vi "Program Blank Device.vi"(0 "State-machine Local Variables":T1={"Message"="", "Homed?"=FALSE, "NextState"=enum."Timeout", "G.Load"=0.0, "G.Position"=0.0, "Load#"=0, "[G.Loads]"=[], "[TotalLoads]"=[], "[Errors]"=[], "ZeroWait"=0, "Results"=[], "DwellWait"=FALSE, "Test Result"=FALSE, "[CondyleLoads]"=[], "[Max]"=[], "[Min]"=[], "Valid String?"=FALSE, "ScanTime"=timestamp(0 s since 1904-01-01), "ScannedString"="", "LabelDevID"=0, "MfgDate"=timestamp(0 s since 1904-01-01), "[EEPROM Cmds]"=[], "[CalData]"=[], "[A/Ds]"=[], "[A/Dmax]"=[], "[A/Dmin]"=[], "BattMax"=0.0, "BattMin"=0.0, "DwellTime"=2000, "PendingDeviceType"="", "Zero G.load"=0.0, "GAINC Value"="", "Programming Step"=enum."Load EEPROM", "Front Panel Program?"=FALSE, "Final Program?"=FALSE, "PCB Score"=100, "AssyScore"=100, "Pass/Fail #"="", "Result String"="", "Programming Mode"=enum."Initial Program", "Angle Test Step"=enum."Initialize", "Accel Values"=[], "Shutdown Counter"=0, "V1"=0, "V2"=0, "V3"=0, "V4"=0, "EEPROM Data"=[], "Counter"=0, "Page#"=0, "Timer"=timestamp(0 s since 1904-01-01), "Use Mark10?"=FALSE, "Eng-Result#"=0, "DUT Serial #"=0, "Scroll Message?"=FALSE, "Clear Message"=FALSE, "Batt Test Step "=enum."Initialize", "RXTX Window Found?"=FALSE, "Shutdown First Call?"=FALSE, "A2 Delay (msec)"=500, "Support Script"={"Script #"="", "Script Revision"="", "[OEMs]"=[], "[[DeviceTypes]]"=[], "[[DeviceTypesVals]]"=[], "[[List of Errors]]"=[], "Default GAINC"="", "[[ASICtrims]]"=[], "ID For Echo"="", "Condyle A CalFactor"=100, "Condyle B CalFactor"=100, "[OEMs Prefix]"=[], "Packet ID 18"="", "[[Force Table Load Test]]"=[], "[[Force Table AccurTest]]"=[]}, "Serial Table"={"Serial File Path"=path "", "[[Serial Lookup Table]]"=[], "Serial Device Info"=[], "Valid Serial?"=FALSE}, "Target Information"={"Target Brand"="", "Target DeviceType"="", "Target Serial#"=100, "Target Lot#"=0, "Target DevID"=0, "Target Channel"=5}, "Operator"="", "COM Port"="", "Config Path"=path "", "Tx Array"=[], "DUT Parameters"={"Channel"=0, "DeviceID"=0, "Script Rev"=0, "Month"=0, "Day"=0, "Year"=0, "Lot#"=0, "V1"=0, "V2"=0, "V3"=0, "V4"=0, "MFG"=0, "Cal FactorA 10"=0, "Cal FactorB 10  "=0, "Cal FactorA 16"=0, "Cal FactorB 16"=0, "ASICtrim"=[], "TmpChan"=0, "GAINC"="", "Brand"="", "Device"="", "Serial #"=0, "Batt310"=0, "Batt 280"=0}, "FTS Main?"=FALSE, "Loading"={"[Forces]"=[], "[Dwell]"=[], "Loading Step"=enum."Initialize Test"}, "Software Version"="", "Correction Factor"="", "Second Load Test"=FALSE, "Acc Loads"=[], "Mark10 Config"={"H2S%"=[80.0, 85.0, 90.0, 95.0, 100.0], "H2S Speed"=[12.0, 8.0, 6.0, 4.0, 2.0], "H to S"=2.0, "Home Speed"=1.0, "LoadWin"=0.0, "Load Speed"=0.0, "PID"={"Kp"=0.04, "Kd"=0.005001, "Ki"=2.9999999999999923e-05}}, "Channels"={"Transceiver Ch"=5, "Operating Ch"=5, "Start Ch"=0}, "Channel EEPROM"=[], "Load Notes"=[], "Engr Log?"=FALSE, "Time"=[], "Program Retry"=FALSE, "Operator Channel"="", "Target Channel "="", "New Data Program"=FALSE, "NFHU Pass?"=FALSE, "Cycle Number"=0, "Cal Cycle#"=0, "[Avg G.Loads] "=[], "[Avg A/Ds] "=[], "Cal Retry?"=FALSE, "[Total A/Ds]  "=[], "Cycle Num LA"=0, "LA Cycle# "=0, "Shim Num"=0, "Shim#  "=0, "Angle Test?"=FALSE} {"Mark10 Config"."PID"."Ki" min=0.0 max=200.0 format="%.6f"; "Mark10 Config"."PID"."Kd" min=0.0 max=200.0 format="%.6f"; "Mark10 Config"."PID"."Kp" min=0.0 max=200.0 format="%.6f"; "DUT Parameters"."ASICtrim" format="%02x"}, 11 "error in (no error)":errorcluster) -> (4 "State-machine Local Variables 2":T1={"Message"="", "Homed?"=FALSE, "NextState"=enum."Timeout", "G.Load"=0.0, "G.Position"=0.0, "Load#"=0, "[G.Loads]"=[], "[TotalLoads]"=[], "[Errors]"=[], "ZeroWait"=0, "Results"=[], "DwellWait"=FALSE, "Test Result"=FALSE, "[CondyleLoads]"=[], "[Max]"=[], "[Min]"=[], "Valid String?"=FALSE, "ScanTime"=timestamp(0 s since 1904-01-01), "ScannedString"="", "LabelDevID"=0, "MfgDate"=timestamp(0 s since 1904-01-01), "[EEPROM Cmds]"=[], "[CalData]"=[], "[A/Ds]"=[], "[A/Dmax]"=[], "[A/Dmin]"=[], "BattMax"=0.0, "BattMin"=0.0, "DwellTime"=2000, "PendingDeviceType"="", "Zero G.load"=0.0, "GAINC Value"="", "Programming Step"=enum."Load EEPROM", "Front Panel Program?"=FALSE, "Final Program?"=FALSE, "PCB Score"=100, "AssyScore"=100, "Pass/Fail #"="", "Result String"="", "Programming Mode"=enum."Initial Program", "Angle Test Step"=enum."Initialize", "Accel Values"=[], "Shutdown Counter"=0, "V1"=0, "V2"=0, "V3"=0, "V4"=0, "EEPROM Data"=[], "Counter"=0, "Page#"=0, "Timer"=timestamp(0 s since 1904-01-01), "Use Mark10?"=FALSE, "Eng-Result#"=0, "DUT Serial #"=0, "Scroll Message?"=FALSE, "Clear Message"=FALSE, "Batt Test Step "=enum."Initialize", "RXTX Window Found?"=FALSE, "Shutdown First Call?"=FALSE, "A2 Delay (msec)"=500, "Support Script"={"Script #"="", "Script Revision"="", "[OEMs]"=[], "[[DeviceTypes]]"=[], "[[DeviceTypesVals]]"=[], "[[List of Errors]]"=[], "Default GAINC"="", "[[ASICtrims]]"=[], "ID For Echo"="", "Condyle A CalFactor"=100, "Condyle B CalFactor"=100, "[OEMs Prefix]"=[], "Packet ID 18"="", "[[Force Table Load Test]]"=[], "[[Force Table AccurTest]]"=[]}, "Serial Table"={"Serial File Path"=path "", "[[Serial Lookup Table]]"=[], "Serial Device Info"=[], "Valid Serial?"=FALSE}, "Target Information"={"Target Brand"="", "Target DeviceType"="", "Target Serial#"=100, "Target Lot#"=0, "Target DevID"=0, "Target Channel"=5}, "Operator"="", "COM Port"="", "Config Path"=path "", "Tx Array"=[], "DUT Parameters"={"Channel"=0, "DeviceID"=0, "Script Rev"=0, "Month"=0, "Day"=0, "Year"=0, "Lot#"=0, "V1"=0, "V2"=0, "V3"=0, "V4"=0, "MFG"=0, "Cal FactorA 10"=0, "Cal FactorB 10  "=0, "Cal FactorA 16"=0, "Cal FactorB 16"=0, "ASICtrim"=[], "TmpChan"=0, "GAINC"="", "Brand"="", "Device"="", "Serial #"=0, "Batt310"=0, "Batt 280"=0}, "FTS Main?"=FALSE, "Loading"={"[Forces]"=[], "[Dwell]"=[], "Loading Step"=enum."Initialize Test"}, "Software Version"="", "Correction Factor"="", "Second Load Test"=FALSE, "Acc Loads"=[], "Mark10 Config"={"H2S%"=[80.0, 85.0, 90.0, 95.0, 100.0], "H2S Speed"=[12.0, 8.0, 6.0, 4.0, 2.0], "H to S"=2.0, "Home Speed"=1.0, "LoadWin"=0.0, "Load Speed"=0.0, "PID"={"Kp"=0.04, "Kd"=0.005001, "Ki"=2.9999999999999923e-05}}, "Channels"={"Transceiver Ch"=5, "Operating Ch"=5, "Start Ch"=0}, "Channel EEPROM"=[], "Load Notes"=[], "Engr Log?"=FALSE, "Time"=[], "Program Retry"=FALSE, "Operator Channel"="", "Target Channel "="", "New Data Program"=FALSE, "NFHU Pass?"=FALSE, "Cycle Number"=0, "Cal Cycle#"=0, "[Avg G.Loads] "=[], "[Avg A/Ds] "=[], "Cal Retry?"=FALSE, "[Total A/Ds]  "=[], "Cycle Num LA"=0, "LA Cycle# "=0, "Shim Num"=0, "Shim#  "=0, "Angle Test?"=FALSE} {"Mark10 Config"."PID"."Ki" min=0.0 max=200.0 format="%.6f"; "Mark10 Config"."PID"."Kd" min=0.0 max=200.0 format="%.6f"; "Mark10 Config"."PID"."Kp" min=0.0 max=200.0 format="%.6f"; "DUT Parameters"."ASICtrim" format="%02x"}, 6 "Program Successful":bool, 15 "error out":errorcluster)   [LabVIEW 2015]
uses:
  Controls/LocalVars.ctl
  Controls/Gen2 FT states.ctl
  Controls/Iniial Device Programming.ctl
  ProgramStageControl.ctl
  Controls/Batt Cap Steps.ctl
  Controls/Support Script.ctl
  Controls/Serial Table.ctl
  Controls/Device Information.ctl
  Controls/InfoPacket.ctl
  Controls/Loading.ctl
  Controls/Load Step.ctl
  Controls/Mark10 Config.ctl
  Controls/PID parameters.ctl
  Controls/Channels.ctl
  Controls/Blank Program State.ctl
  RxTx/XceiverStates.ctl
  RxTx/XceiverCmds.ctl
  Controls/Gen2 FT Globals.vi
panel:
  out "Numeric":i32
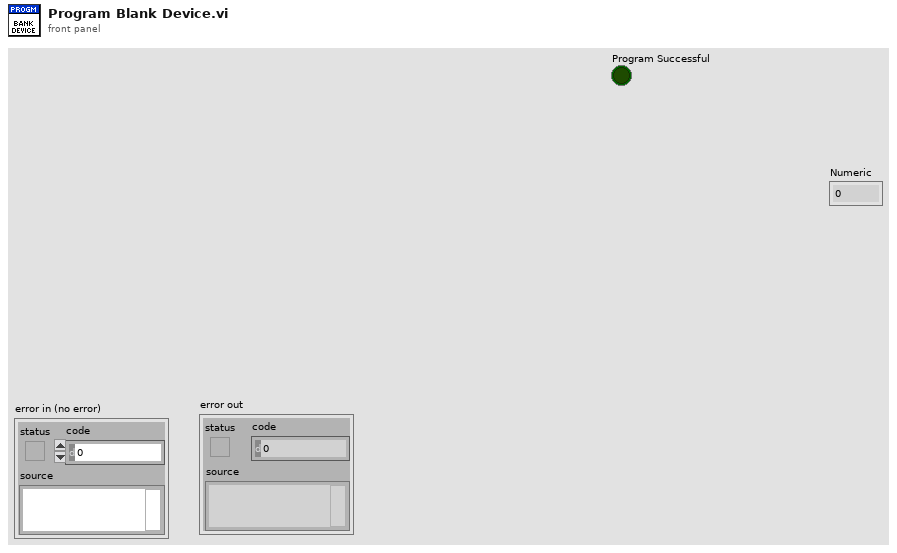
[diagram p1: front panel]
types:
  T1 = typedef "LocalVars.ctl" = cluster{"Message":string, "Homed?":bool, "NextState":T2, "G.Load":dbl, "G.Position":dbl, "Load#":i32, "[G.Loads]":dbl[], "[TotalLoads]":dbl[], "[Errors]":dbl[][], "ZeroWait":u32, "Results":dbl[], "DwellWait":bool, "Test Result":bool, "[CondyleLoads]":dbl[][], "[Max]":dbl[], "[Min]":dbl[], "Valid String?":bool, "ScanTime":timestamp, "ScannedString":string, "LabelDevID":u32, "MfgDate":timestamp, "[EEPROM Cmds]":u8[][], "[CalData]":u8[][], "[A/Ds]":dbl[][], "[A/Dmax]":dbl[], "[A/Dmin]":dbl[], "BattMax":dbl, "BattMin":dbl, "DwellTime":i32, "PendingDeviceType":string, "Zero G.load":dbl, "GAINC Value":string, "Programming Step":T3, "Front Panel Program?":bool, "Final Program?":bool, "PCB Score":i32, "AssyScore":i32, "Pass/Fail #":string, "Result String":string, "Programming Mode":T4, "Angle Test Step":enum16{"Initialize", "Get X", "Get Y", "Get Z", "Next Test"}, "Accel Values":dbl[][], "Shutdown Counter":u32, "V1":i32, "V2":i32, "V3":i32, "V4":i32, "EEPROM Data":i32[][], "Counter":i32, "Page#":i32, "Timer":timestamp, "Use Mark10?":bool, "Eng-Result#":u32, "DUT Serial #":i32, "Scroll Message?":bool, "Clear Message":bool, "Batt Test Step ":T5, "RXTX Window Found?":bool, "Shutdown First Call?":bool, "A2 Delay (msec)":i16, "Support Script":T6, "Serial Table":T7, "Target Information":T8, "Operator":string, "COM Port":string, "Config Path":path, "Tx Array":u8[], "DUT Parameters":T9, "FTS Main?":bool, "Loading":T10, "Software Version":string, "Correction Factor":string, "Second Load Test":bool, "Acc Loads":dbl[][], "Mark10 Config":T12, "Channels":T14, "Channel EEPROM":i32[][], "Load Notes":string[], "Engr Log?":bool, "Time":timestamp[], "Program Retry":bool, "Operator Channel":string, "Target Channel ":string, "New Data Program":bool, "NFHU Pass?":bool, "Cycle Number":i32, "Cal Cycle#":i32, "[Avg G.Loads] ":dbl[], "[Avg A/Ds] ":dbl[][], "Cal Retry?":bool, "[Total A/Ds]  ":dbl[][], "Cycle Num LA":i32, "LA Cycle# ":i32, "Shim Num":i32, "Shim#  ":i32, "Angle Test?":bool}
  T2 = typedef "Gen2 FT states.ctl" = enum16{"---------SETUP-------", "Initialization", "Read Support Data", "Initialize Mark-10", "Initialize Transceiver", "------UTILITIES------", "Change DUT Channel", "Find RxTx Window", "Reset Device", "Scan Channels", "Read Serial Lookup", "Shutdown Device", "ESTOP", "--------USER---------", "Timeout", "-----PROGRAM-----", "Program Device", "------MARK10--------", "Go Home", "MoveUp", "MoveDown", "Goto Load", "Goto Position", "Stop Motor", "---------TESTS--------", "Start Test", "Angle Test", "Load Test", "Load Accuracy Test", "Battery Test", "------RESULTS-------", "End Test", "Display Result", "--------EXIT--------", "Exit"}
  T3 = typedef "Iniial Device Programming.ctl" = enum16{"Load EEPROM", "Send First A1", "Send EEPROM", "Send A1", "Check EEPROM Echo", "Verify transmission", "Programming Successful", "Programming Failed"}
  T4 = typedef "ProgramStageControl.ctl" = enum16{"Initial Program", "GainC", "Scales"}
  T5 = typedef "Batt Cap Steps.ctl" = enum16{"Initialize", "Collect 2.8 Volts", "Collect 3.1 Volts", "Check Results"}
  T6 = typedef "Support Script.ctl" = cluster{"Script #":string, "Script Revision":string, "[OEMs]":string[], "[[DeviceTypes]]":string[][], "[[DeviceTypesVals]]":u16[][], "[[List of Errors]]":string[][], "Default GAINC":string, "[[ASICtrims]]":u8[][], "ID For Echo":string, "Condyle A CalFactor":i32, "Condyle B CalFactor":i32, "[OEMs Prefix]":string[], "Packet ID 18":string, "[[Force Table Load Test]]":dbl[][], "[[Force Table AccurTest]]":dbl[][]}
  T7 = typedef "Serial Table.ctl" = cluster{"Serial File Path":path, "[[Serial Lookup Table]]":string[][], "Serial Device Info":string[], "Valid Serial?":bool}
  T8 = typedef "Device Information.ctl" = cluster{"Target Brand":string, "Target DeviceType":string, "Target Serial#":i32, "Target Lot#":u32, "Target DevID":u32, "Target Channel":u8}
  T9 = typedef "InfoPacket.ctl" = cluster{"Channel":u8, "DeviceID":u32, "Script Rev":u8, "Month":u8, "Day":u8, "Year":u8, "Lot#":u32, "V1":u16, "V2":u16, "V3":u16, "V4":u16, "MFG":u8, "Cal FactorA 10":u8, "Cal FactorB 10  ":u8, "Cal FactorA 16":u8, "Cal FactorB 16":u8, "ASICtrim":u8[], "TmpChan":u8, "GAINC":string, "Brand":string, "Device":string, "Serial #":u64, "Batt310":u16, "Batt 280":u16}
  T10 = typedef "Loading.ctl" = cluster{"[Forces]":dbl[], "[Dwell]":dbl[], "Loading Step":T11}
  T11 = typedef "Load Step.ctl" = enum16{"Initialize Test", "Go Home", "Detect Dev Surface", "Wait to zero Device", "Zero Device", "Do Test", "Test Result"}
  T12 = typedef "Mark10 Config.ctl" = cluster{"H2S%":dbl[], "H2S Speed":dbl[], "H to S":dbl, "Home Speed":dbl, "LoadWin":dbl, "Load Speed":dbl, "PID":T13}
  T13 = typedef "PID parameters.ctl" = cluster{"Kp":dbl, "Kd":dbl, "Ki":dbl}
  T14 = typedef "Channels.ctl" = cluster{"Transceiver Ch":u8, "Operating Ch":u8, "Start Ch":u8}
  T15 = typedef "Blank Program State.ctl" = enum16{"Loading EEPROM data", "Send Page 0", "Program", "Verify transmission", "Programming Successful", "Programming Failed"}
  T16 = typedef "XceiverStates.ctl" = enum16{"Initialize", "Rx", "Tx", "Raw Mode", "Clear Buffer", "ClearEcho", "Read Buffer", "Close"}
  T17 = typedef "XceiverCmds.ctl" = enum8{"Get Window", "Set Window", "Load&Xmit", "Find Window", "Load CC1101", "Blink LED1", "Blink LED2", "Gen2 Mode", "Request Rev", "Gen2 Mode & Req Rev", "Load Device Settings", "Reset Xceiver", "Set Channel", "Read Channel"}
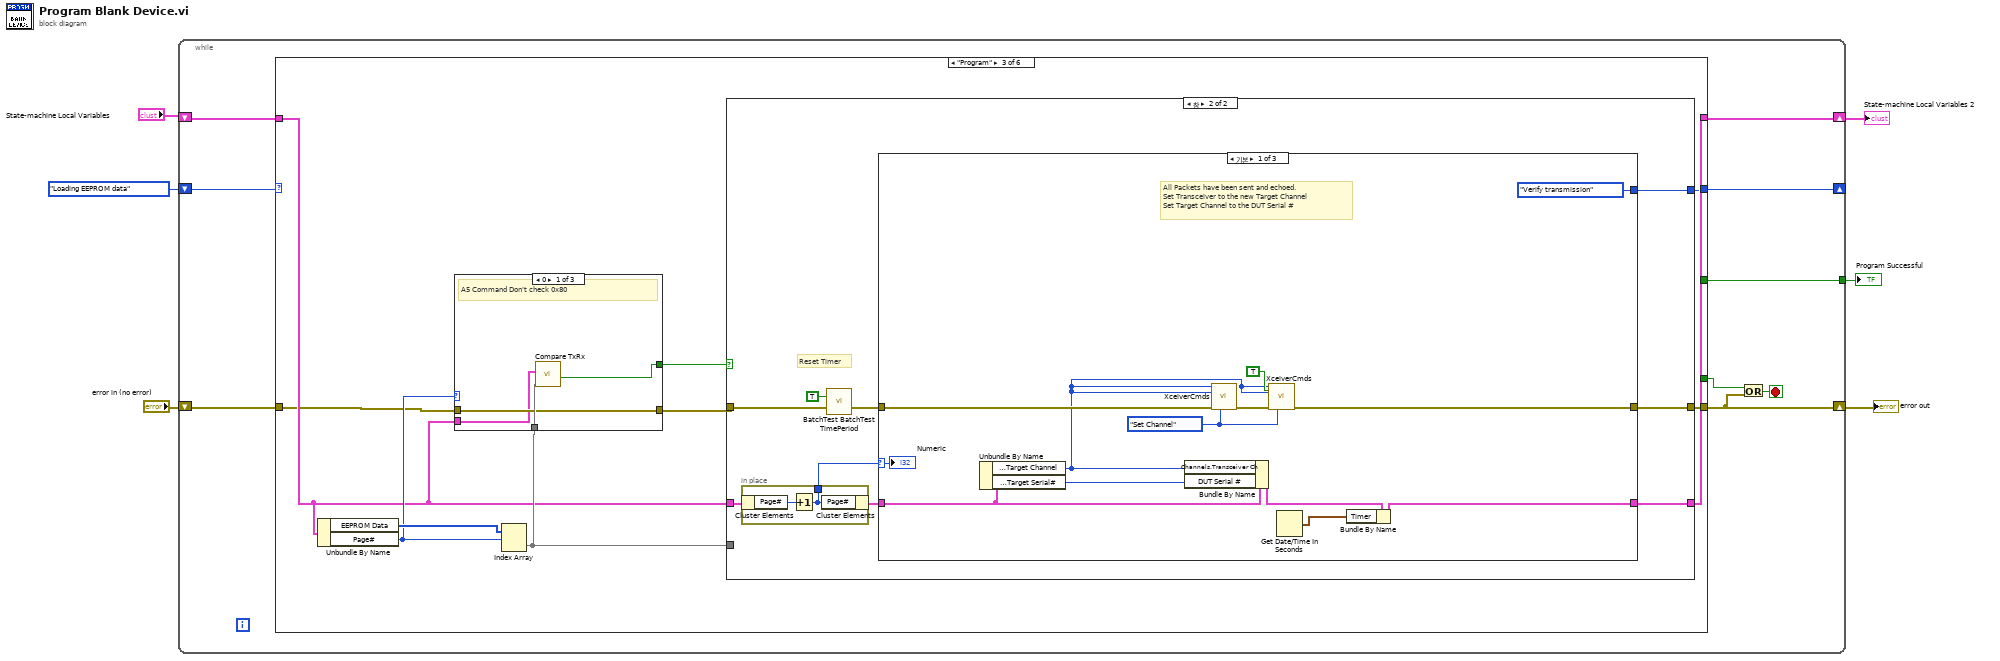
[diagram p0: block diagram]
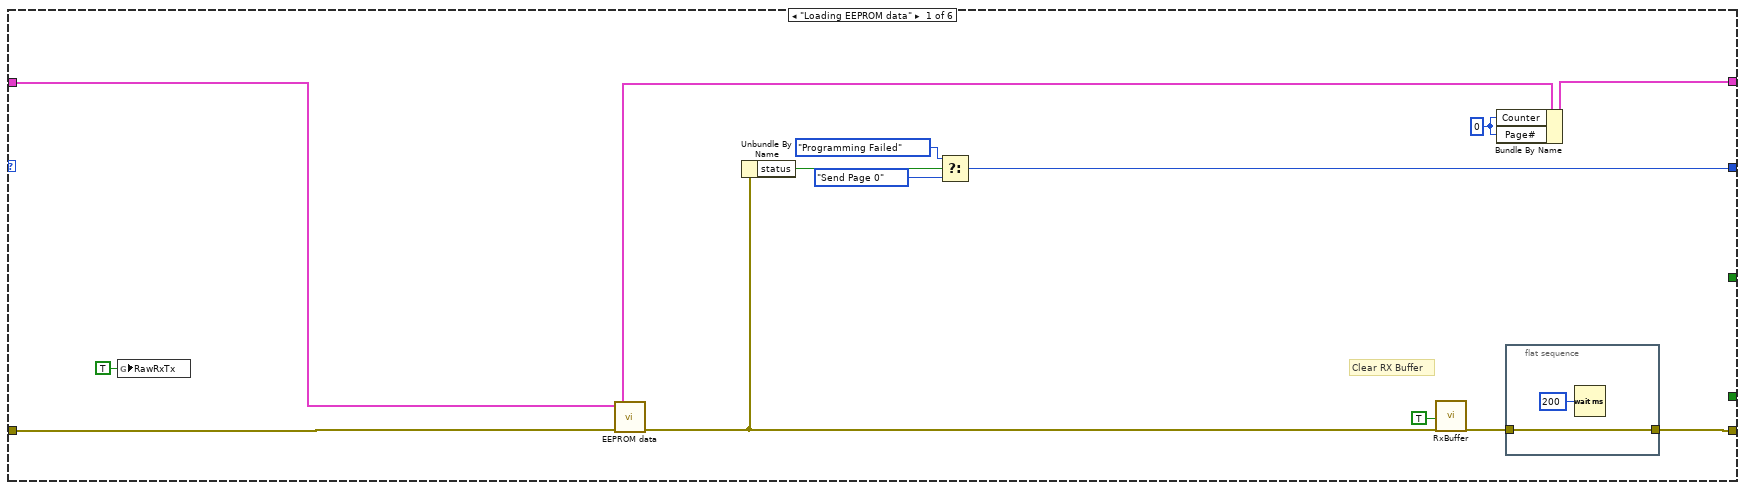
[diagram p2: hidden frame]
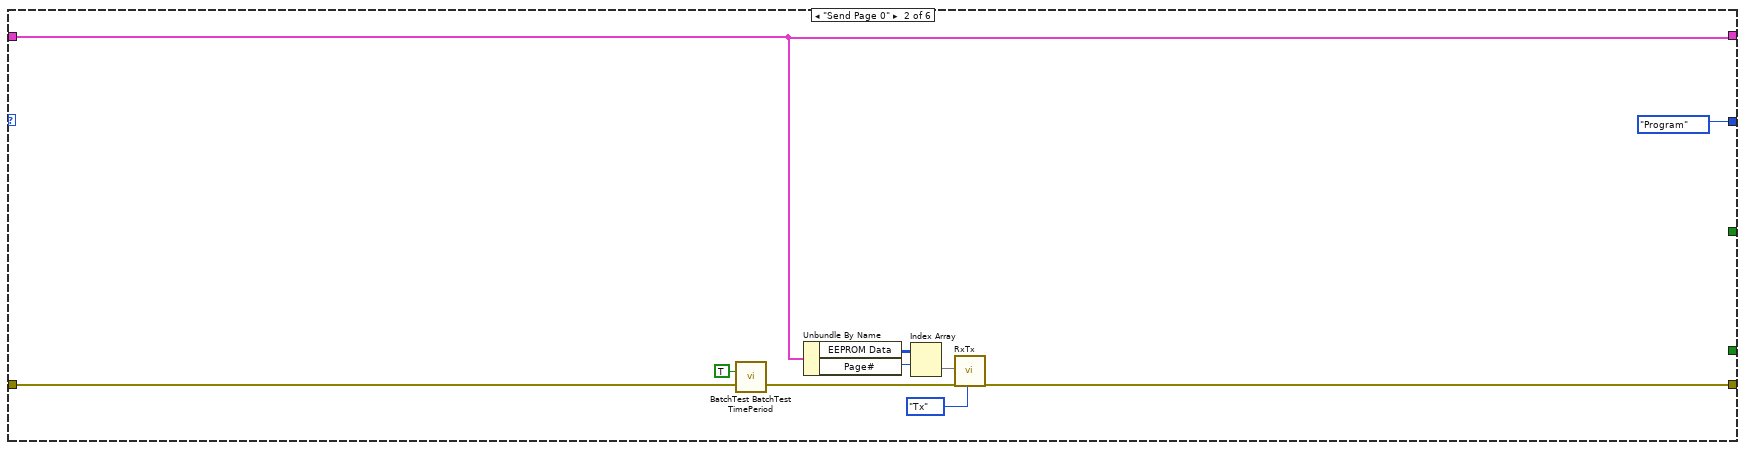
[diagram p3: hidden frame]
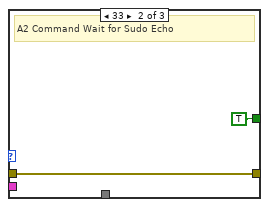
[diagram p4: hidden frame]
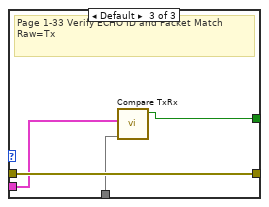
[diagram p5: hidden frame]
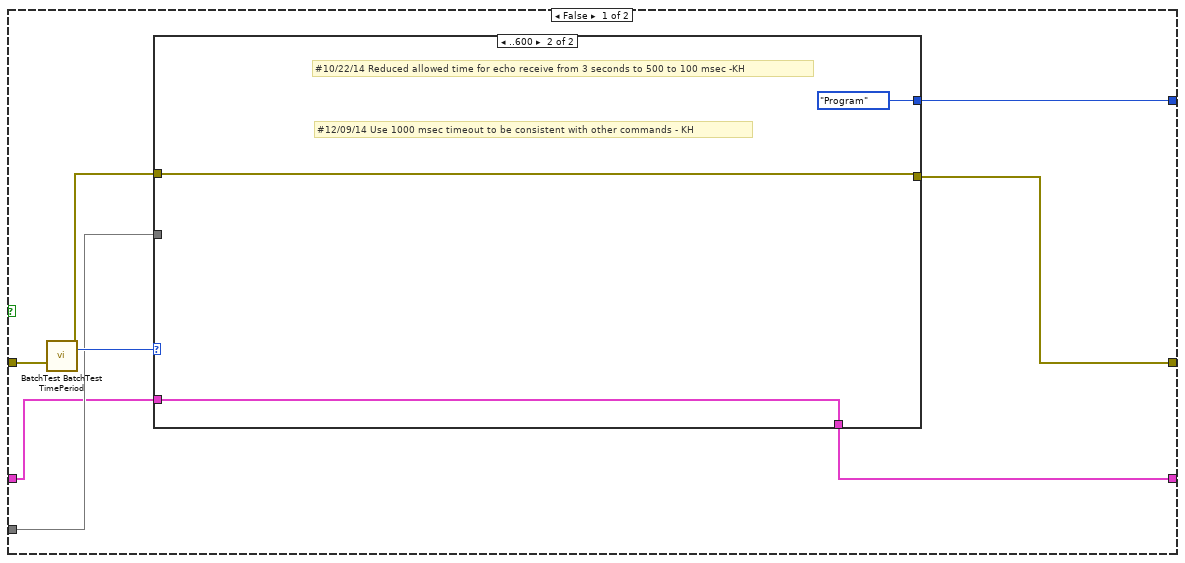
[diagram p6: hidden frame]
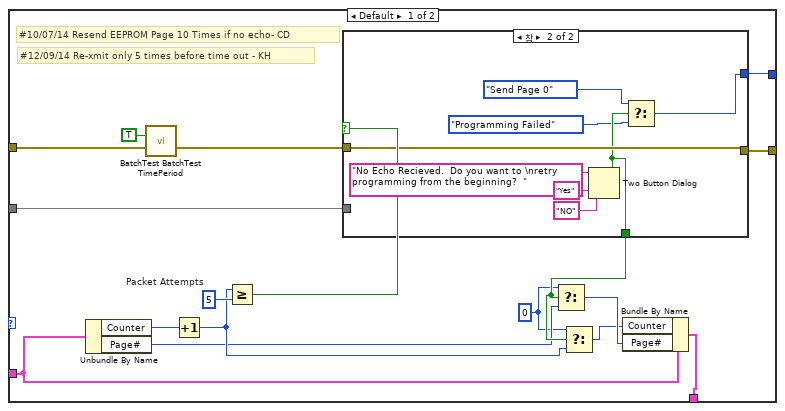
[diagram p7: hidden frame]
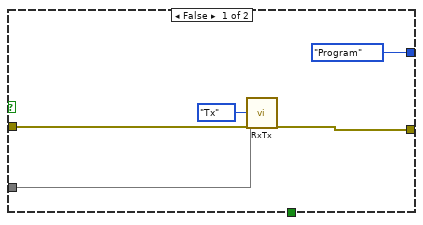
[diagram p8: hidden frame]
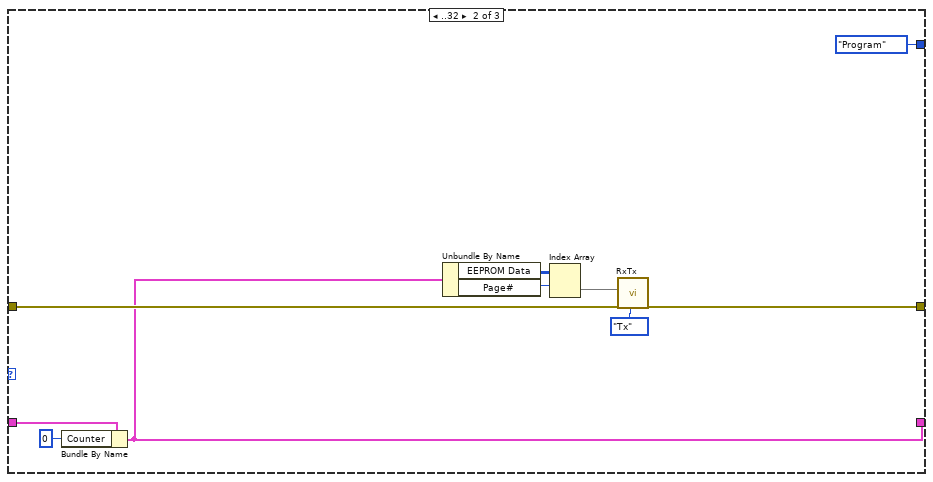
[diagram p9: hidden frame]
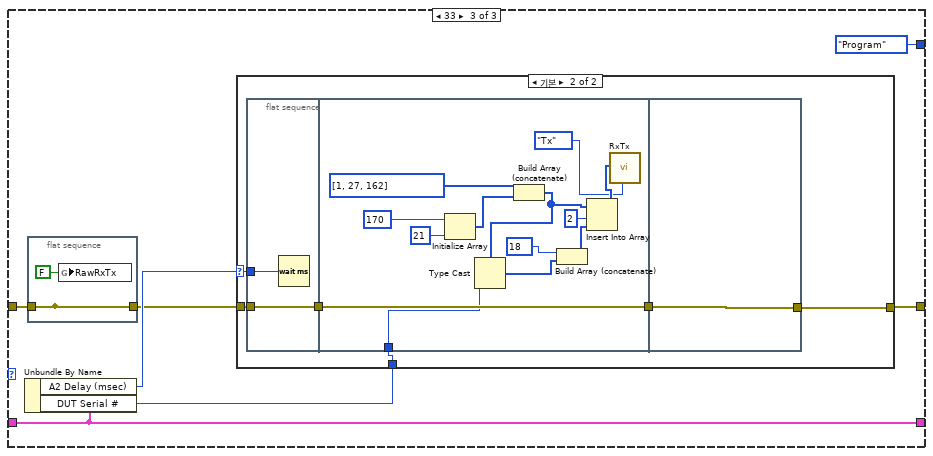
[diagram p10: hidden frame]
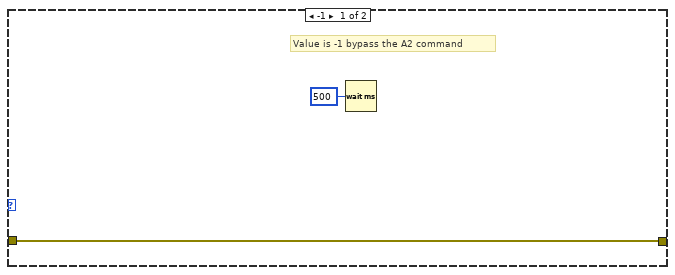
[diagram p11: hidden frame]
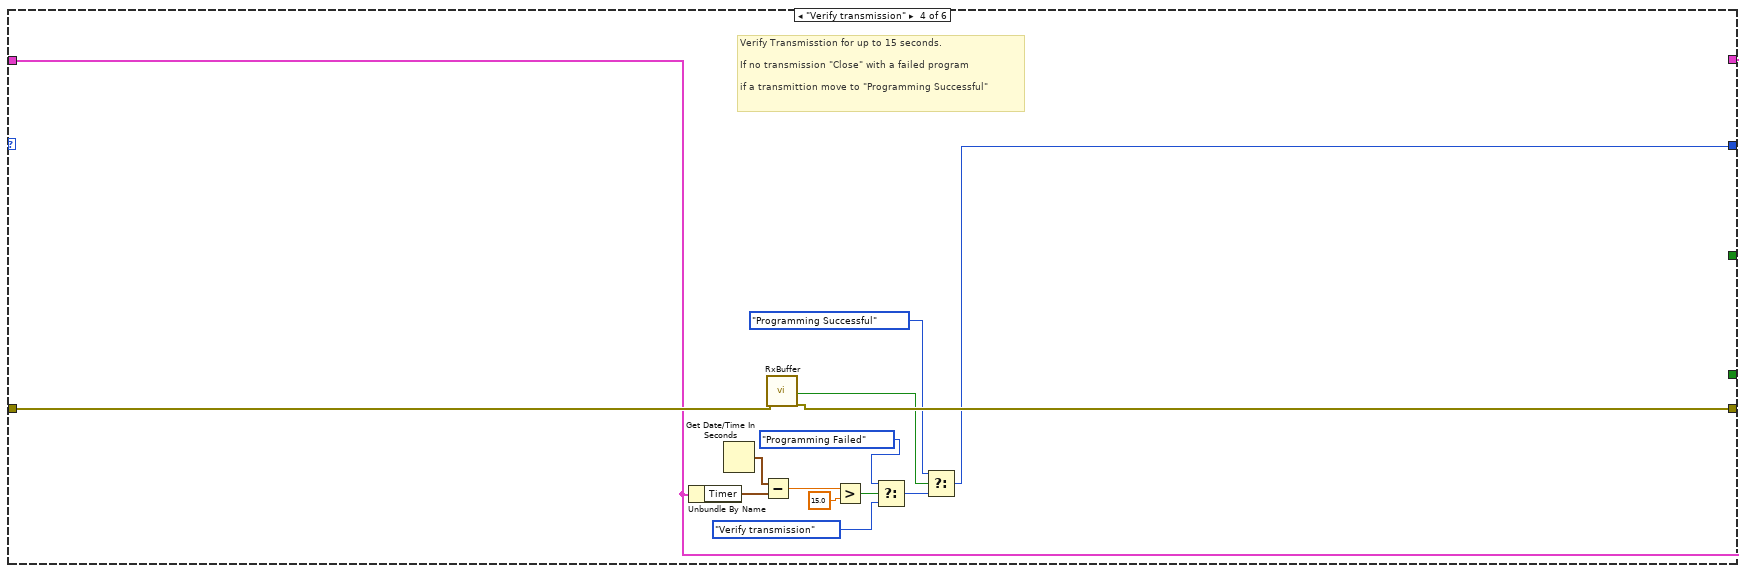
[diagram p12: hidden frame]
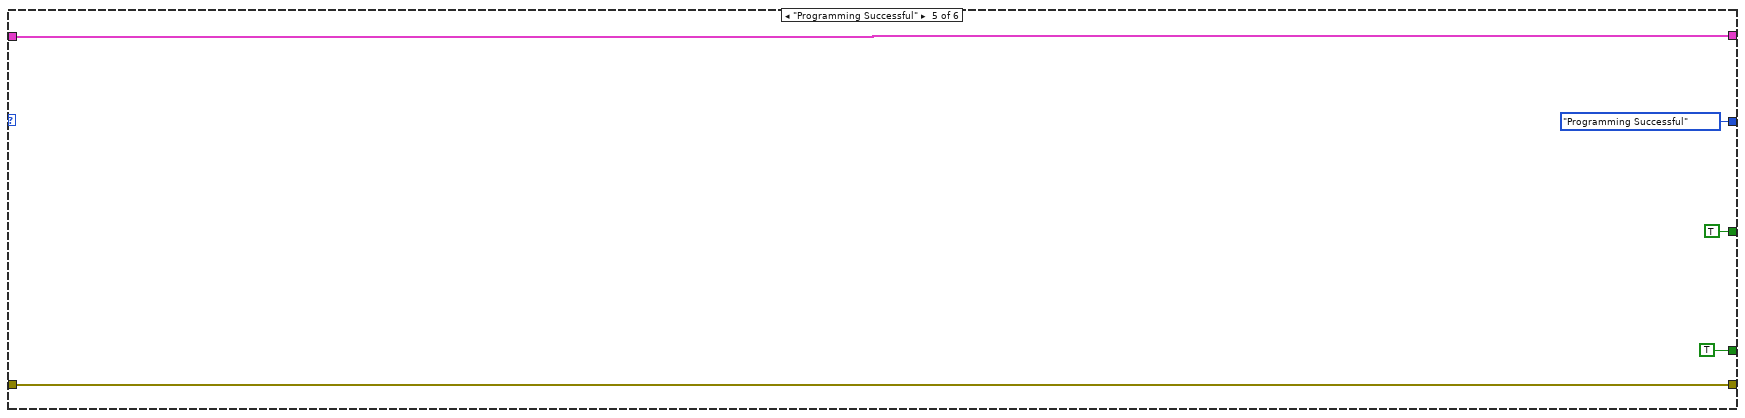
[diagram p13: hidden frame]
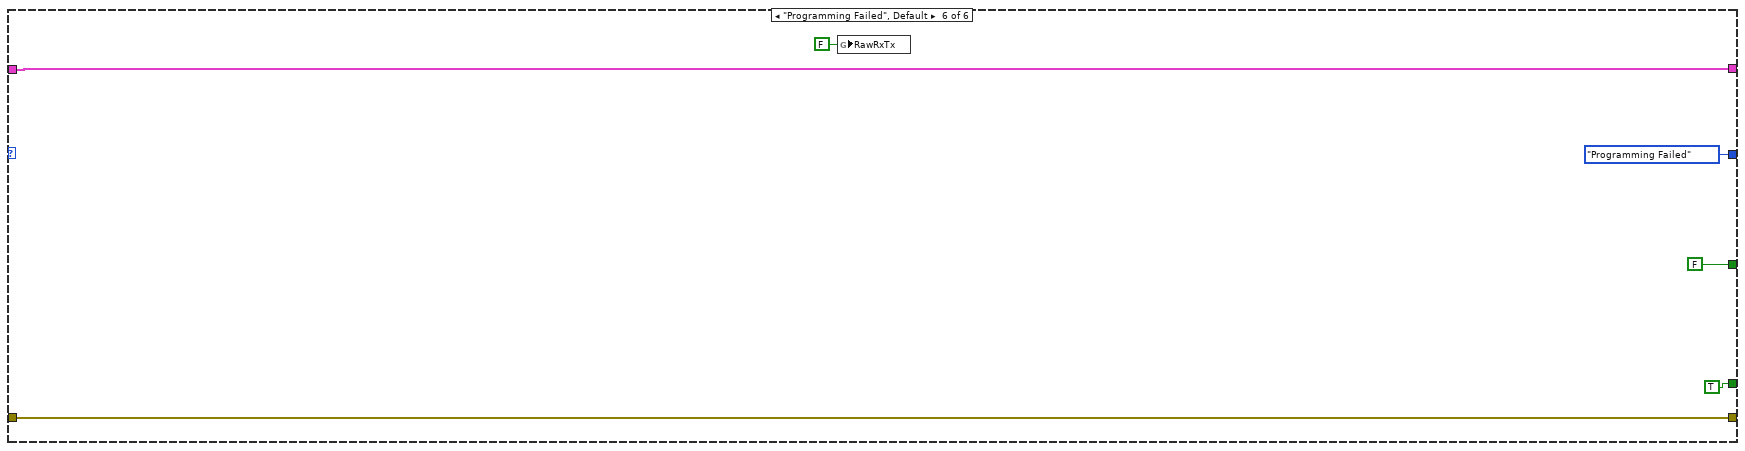
[diagram p14: hidden frame]
diagram:
  n1 = while {
    shift-right: [w11] -> w5
    shift-left: "error in (no error)" -> [w15]
    shift-right: [w13] -> w3
    shift-left: "State-machine Local Variables" -> [w14]
    shift-right: [w8] -> _
    shift-left: Blank_Program_State."Loading EEPROM data" ("t") -> [w9]
    tunnel: [w7] -> w1
    stop <- w10 stop-if-true
    n2 = case shown="\"Program\"" w9 {
      tunnel: [w17 w40 w50 w182 w186 w191] -> w11
      tunnel: w15 -> [w25 w32 w41 w181 w186 w191]
      tunnel: [_ _ _ _ TRUE TRUE] -> w12
      tunnel: [w28 w33 w44 w174 w185 w190] -> w13
      tunnel: w14 -> [w27 w33 w42 w174 w185 w190]
      tunnel: [w18 Blank_Program_State."Program" ("t") w43 w169 Blank_Program_State."Programming Successful" ("t") Blank_Program_State."Programming Failed" ("t")] -> w8
      tunnel: [_ _ _ _ TRUE FALSE] -> w7
      frame "Loading EEPROM data" {
        w24 = 0 ("Counter")
        # "Clear RX Buffer"
        n3 = global write "Gen2 FT Globals.vi" "RawRxTx"(TRUE ("Initialize?")) -> ()
        n4 = call "EEPROM data.vi"("error in (no error)"=w25, "State-machine Local Variables"=w27) -> ("error out"=w21:errorcluster, "State-machine Local Variables 2"=w26:T1)  [unwired: 8 in]
        n5 = Unbundle By Name(w21) -> ("status"=w29:bool)
        n6 = Select(t=Blank_Program_State."Programming Failed", s=w29, f=Blank_Program_State."Send Page 0" ("t")) -> (s? t:f=w18:T15)
        n7 = call "RxBuffer.vi"("Clear?"=TRUE, "error in (no error)"=w21) -> ("error out"=w16:errorcluster)  [unwired: 6 in, 11 out]
        n8 = Bundle By Name(cluster=w26, "Counter"=w24, "Page#"=w24) -> (w28:T1)
        n9 = flat-sequence {
          tunnel: [w31] -> w17
          tunnel: w16 -> [w31]
          frame #0 {
            n10 = Wait (ms)(milliseconds to wait=u32 200) -> ()  [unwired: 1 out]
          }
        }
      }
      frame "Send Page 0" {
        n11 = call "BatchTest BatchTest TimePeriod.vi"("Initialize?"=TRUE) -> ()  [unwired: 13 in, 2 out]
        n12 = Unbundle By Name(w33) -> ("EEPROM Data"=w38:i32[][], "Page#"=w37:i32)
        n13 = Index Array(array=w38, index (row)=w37) -> (element=w35:i32[])  [unwired: 1 in]
        n14 = call "RxTx.vi"("[TxData]"=w35, "error in (no error)"=w32, "Action"=XceiverStates."Tx") -> ("error out"=w40:errorcluster)  [unwired: 8 in, 8 out]
      }
      frame "Program" {
        n15 = Unbundle By Name(w42) -> ("EEPROM Data"=w49:i32[][], "Page#"=w47:i32)
        n16 = Index Array(array=w49, index (row)=w47) -> (element=w46:i32[])  [unwired: 1 in]
        n17 = case shown="0" w47 {
          tunnel: [w51 TRUE ("Match?") w58] -> w48
          tunnel: w46 -> [w54 _ w59]
          tunnel: w41 -> [w53 w56 w60]
          tunnel: [w53 w56 w60] -> w45
          tunnel: w42 -> [w52 _ w57]
          frame 0 {
            # "A5 Command Don't check 0x80"
            n18 = call "Compare TxRx.vi"("RawTx"=w54, "Data Cluster In"=w52) -> ("Content?"=w51:bool)  [unwired: 7 in, 2 out]
          }
          frame 33 {
            # "A2 Command Wait for Sudo Echo"
          }
          frame Default {
            # "Page 1-33 Verify ECHO ID and Packet Match\nRaw=Tx"
            n19 = call "Compare TxRx.vi"("RawTx"=w59, "Data Cluster In"=w57) -> ("0x80 + Content?"=w58:bool)  [unwired: 7 in, 2 out]
          }
        }
        n20 = case shown="참" w48 {
          tunnel: [w67 w108] -> w50
          tunnel: w45 -> [w68 w110]
          tunnel: w42 -> [w63 w109]
          tunnel: [w62 w107] -> w44
          tunnel: w46 -> [w64 _]
          tunnel: [w61 w102] -> w43
          frame False {
            n21 = call "BatchTest BatchTest TimePeriod.vi"("error in (no error)"=w68) -> ("Time(mS)"=w65:u32, "error out"=w66:errorcluster)  [unwired: 13 in]
            n22 = case shown="..600" w65 {
              tunnel: [w85 w101] -> w67
              tunnel: w66 -> [w78 w101]
              tunnel: w64 -> [w84 _]
              tunnel: w63 -> [w83 w100]
              tunnel: [w82 w100] -> w62
              tunnel: [w69 Blank_Program_State."Program" ("t")] -> w61
              frame Default {
                w70 = 0 ("Page#")
                w80 = 5  # Packet Attempts
                # "#12/09/14 Re-xmit only 5 times before time out - KH"
                # "#10/07/14 Resend EEPROM Page 10 Times if no echo- CD"
                n23 = Unbundle By Name(w83) -> ("Counter"=w81:i32, "Page#"=w71:i32)
                n24 = call "BatchTest BatchTest TimePeriod.vi"("Initialize?"=TRUE, "error in (no error)"=w78) -> ("error out"=w77:errorcluster)  [unwired: 12 in, 1 out]
                n25 = Increment(x=w81) -> (x+1=w73:i32)
                n26 = Greater Or Equal?(x=w73, y=w80) -> (x >= y?=w79:bool)
                n27 = case shown="참" w79 {
                  tunnel: w77 -> [w89 w98]
                  tunnel: [w88 w98] -> w85
                  tunnel: w84 -> [w87 _]
                  tunnel: [_ w94] -> w74
                  tunnel: [Blank_Program_State."Program" ("t") w92] -> w69
                  frame False {
                    n28 = call "RxTx.vi"("[TxData]"=w87, "error in (no error)"=w89, "Action"=XceiverStates."Tx") -> ("error out"=w88:errorcluster)  [unwired: 8 in, 8 out]
                  }
                  frame True {
                    n29 = Two Button Dialog(message="No Echo Recieved.  Do you want to \nretry programming from the beginning?  ", 1:"NO" ("F button name (\"Cancel\")"), 2:"Yes" ("T button name (\"OK\")")) -> (T button?=w94:bool)
                    n30 = Select(t=Blank_Program_State."Send Page 0", s=w94, f=Blank_Program_State."Programming Failed" ("t")) -> (s? t:f=w92:T15)
                  }
                }
                n31 = Select(t=w70, s=w74, f=w71) -> (s? t:f=w75:i32)
                n32 = Select(t=w70, s=w74, f=w73) -> (s? t:f=w72:i32)
                n33 = Bundle By Name(cluster=w83, "Counter"=w72, "Page#"=w75) -> (w82:T1)
              }
              frame ..600 {
                # "#12/09/14 Use 1000 msec timeout to be consistent with other commands - KH"
                # "#10/22/14 Reduced allowed time for echo receive from 3 seconds to 500 to 100 msec -KH"
              }
            }
          }
          frame True {
            # "Reset Timer"
            n34 = in-place {
              in-place-border: [w167] -> w104
              n35 = in-place-cluster #1(w109) -> ("Page#"=w168:i32)
              n36 = Increment(x=w168) -> (x+1=w167:i32)
              n37 = in-place-cluster #1("Page#"=w167) -> (w105:T1)
            }
            n38 = call "BatchTest BatchTest TimePeriod.vi"("Initialize?"=TRUE, "error in (no error)"=w110) -> ("error out"=w106:errorcluster)  [unwired: 12 in, 1 out]
            n39 = case shown="기본" w104 {
              selector: w104 -> [w123 _ _]
              tunnel: w106 -> [w121 w132 w136]
              tunnel: [w117 w131 w138] -> w108
              tunnel: w105 -> [w122 w130 w139]
              tunnel: [w120 w126 w139] -> w107
              tunnel: [Blank_Program_State."Verify transmission" ("t") Blank_Program_State."Program" ("t") Blank_Program_State."Program" ("t")] -> w102
              frame Default {
                w118 = TRUE ("RF Chip0 Enable")
                w116 = XceiverCmds."Set Channel" ("XceiverCmd")
                # "All Packets have been sent and echoed.\nSet Transceiver to the new Target Channel\nSet Target Channel to the DUT Serial #"
                n40 = Unbundle By Name(w122) -> ("Target Information.Target Channel"=w111:u8, "Target Information.Target Serial#"=w113:i32)
                n41 = Bundle By Name(cluster=w122, "Channels.Transceiver Ch"=w111, "DUT Serial #"=w113) -> (w114:T1)
                n42 = call "XceiverCmds.vi"("RF Chip0 Channel"=w111, "RF Chip1 Channel"=w111, "error in (no error)"=w121, "XceiverCmd"=w116) -> ("error out"=w115:errorcluster)  [unwired: 9 in, 2 out]
                n43 = call "XceiverCmds.vi"("RF Chip0 Channel"=w111, "RF Chip0 Enable"=w118, "RF Chip1 Enable"=w118, "RF Chip1 Channel"=w111, "error in (no error)"=w115, "XceiverCmd"=w116) -> ("error out"=w117:errorcluster)  [unwired: 7 in, 2 out]
                n44 = Get Date/Time In Seconds() -> (seconds since 1Jan1904=w119:timestamp)
                n45 = Bundle By Name(cluster=w114, "Timer"=w119) -> (w120:T1)
                "Numeric" <- w123
              }
              frame ..32 {
                n46 = Bundle By Name(cluster=w130, "Counter"=0) -> (w126:T1)
                n47 = Unbundle By Name(w126) -> ("EEPROM Data"=w129:i32[][], "Page#"=w128:i32)
                n48 = Index Array(array=w129, index (row)=w128) -> (element=w127:i32[])  [unwired: 1 in]
                n49 = call "RxTx.vi"("[TxData]"=w127, "error in (no error)"=w132, "Action"=XceiverStates."Tx") -> ("error out"=w131:errorcluster)  [unwired: 8 in, 8 out]
              }
              frame 33 {
                n50 = Unbundle By Name(w139) -> ("A2 Delay (msec)"=w137:i16, "DUT Serial #"=w140:i32)
                n51 = flat-sequence {
                  tunnel: w136 -> [w141]
                  tunnel: [w141] -> _
                  tunnel: [w141] -> w135
                  frame #0 {
                    n52 = global write "Gen2 FT Globals.vi" "RawRxTx"(FALSE ("RawRxTx")) -> ()
                  }
                }
                n53 = case shown="기본" w137 {
                  selector: w137 -> [_ w146]
                  tunnel: w135 -> [w143 w149]
                  tunnel: w140 -> [_ w148]
                  tunnel: [w143 w147] -> w138
                  frame -1 {
                    # "Value is -1 bypass the A2 command"
                    n54 = Wait (ms)(milliseconds to wait=u32 500) -> ()  [unwired: 1 out]
                  }
                  frame Default {
                    n55 = flat-sequence {
                      tunnel: w149 -> [w152]
                      tunnel: [w152] -> w150
                      tunnel: w146 -> [w151]
                      tunnel: [w165] -> w145
                      tunnel: w150 -> [w165]
                      tunnel: w148 -> [w164]
                      tunnel: [w166] -> w147
                      tunnel: w145 -> [w166]
                      frame #0 {
                        n56 = Wait (ms)(milliseconds to wait=w151) -> ()  [unwired: 1 out]
                      }
                      frame #1 {
                        n57 = Initialize Array(u8 170, 21 ("dimension size")) -> (w160:u8[])
                        n58 = Build Array (concatenate)(u8[] [1, 27, 162] ("initialized array"), w160) -> (w161:u8[])
                        n59 = Type Cast(type=w161, x=w164) -> (*(type *) &x=w159:u8[])
                        n60 = Build Array (concatenate)(u8 18, w159) -> (w163:u8[])
                        n61 = Insert Into Array(array=w161, index=2, new element=w163) -> (w155:u8[])
                        n62 = call "RxTx.vi"("[TxData]"=w155, "Action"=XceiverStates."Tx") -> ()  [unwired: 9 in, 9 out]
                      }
                      frame #2 {
                      }
                    }
                  }
                }
              }
            }
          }
        }
      }
      frame "Verify transmission" {
        # "Verify Transmisstion for up to 15 seconds. \n\nIf no transmission \"Close\" with a failed program\n\nif a transmittion move to \"Programming Successful\""
        n63 = Unbundle By Name(w174) -> ("Timer"=w175:timestamp)
        n64 = Get Date/Time In Seconds() -> (seconds since 1Jan1904=w179:timestamp)
        n65 = Subtract(x=w179, y=w175) -> (x-y=w177:dbl)
        n66 = call "RxBuffer.vi"("error in (no error)"=w181) -> ("New Data"=w173:bool, "error out"=w182:errorcluster)  [unwired: 7 in, 10 out]
        n67 = Greater?(x=w177, y=15.0) -> (0:w176:bool)
        n68 = Select(t=Blank_Program_State."Programming Failed", s=w176, f=Blank_Program_State."Verify transmission" ("t")) -> (s? t:f=w180:T15)
        n69 = Select(t=Blank_Program_State."Programming Successful", s=w173, f=w180) -> (s? t:f=w169:T15)
      }
      frame "Programming Successful" {
      }
      frame "Programming Failed", Default {
        n70 = global write "Gen2 FT Globals.vi" "RawRxTx"(FALSE ("RawRxTx")) -> ()
      }
    }
    n71 = Or(x=w12, y=w11) -> (x .or. y?=w10:bool)
  }
  "error out" <- w5
  "State-machine Local Variables 2" <- w3
  "Program Successful" <- w1
